vi "Template.Utility VI with Q Interface.vi"(7 "Q.Parent":refnum<queue>, 11 "Name":string) -> ()   [LabVIEW 2018]
uses:
  <vilib>/KATE/Queues/Q.Element.ctl
  <vilib>/KATE/Queues/Queue Utils.lvlib
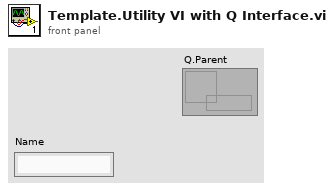
[diagram p1: front panel]
types:
  T1 = cluster{"Q.Parent":refnum<queue>, "Data1":bool, "Data2":string}
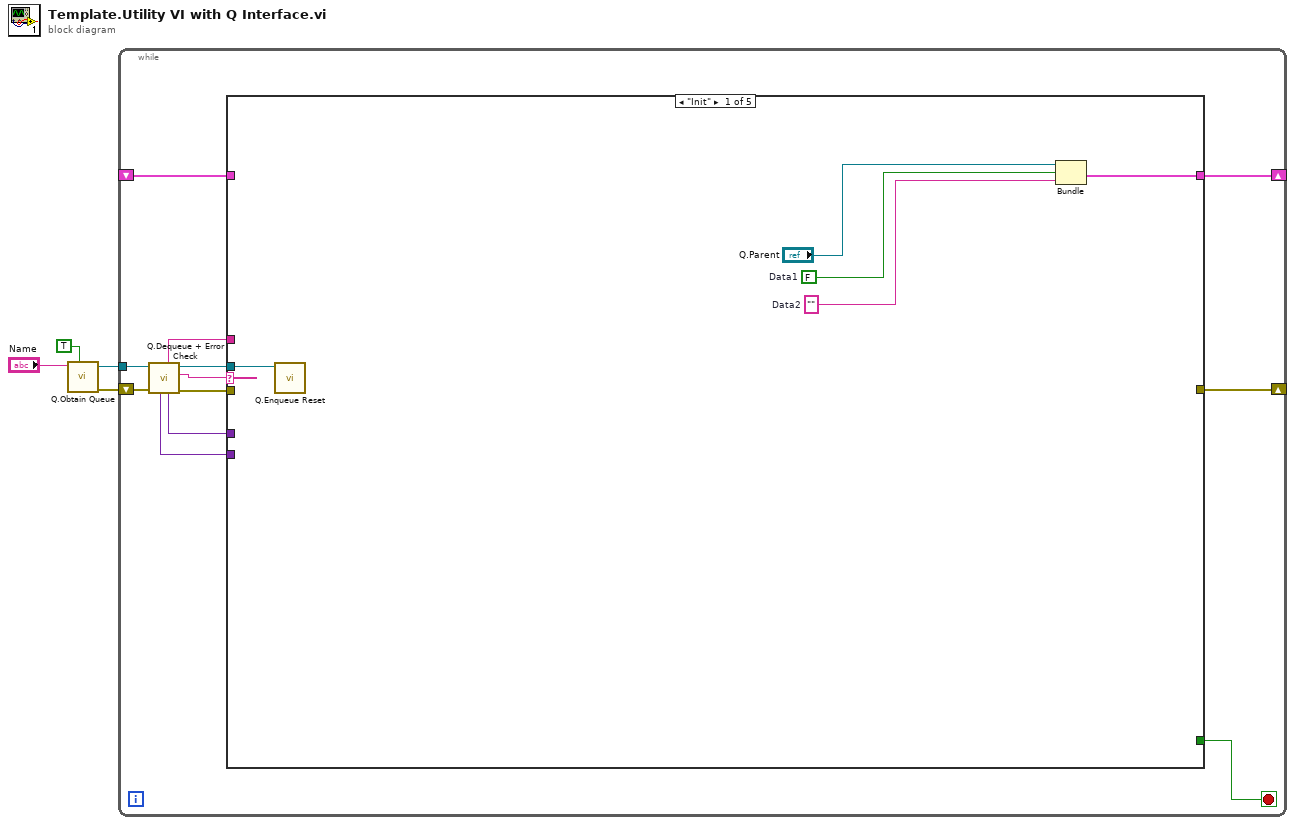
[diagram p0: block diagram]
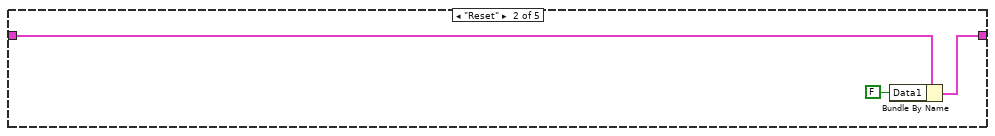
[diagram p2: hidden frame]
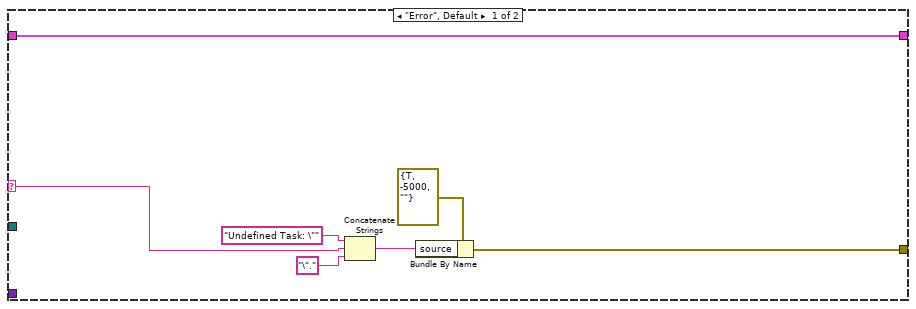
[diagram p4: hidden frame]
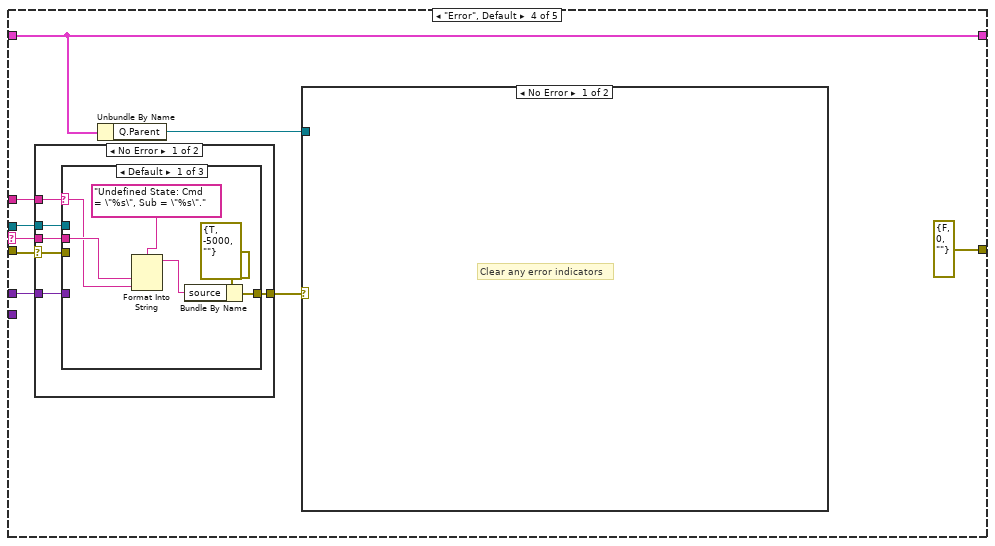
[diagram p5: hidden frame]
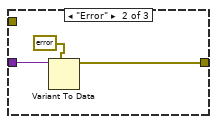
[diagram p6: hidden frame]
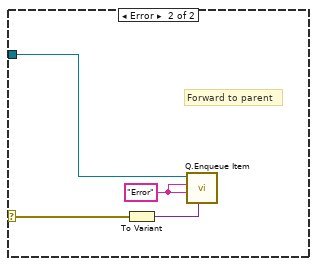
[diagram p9: hidden frame]
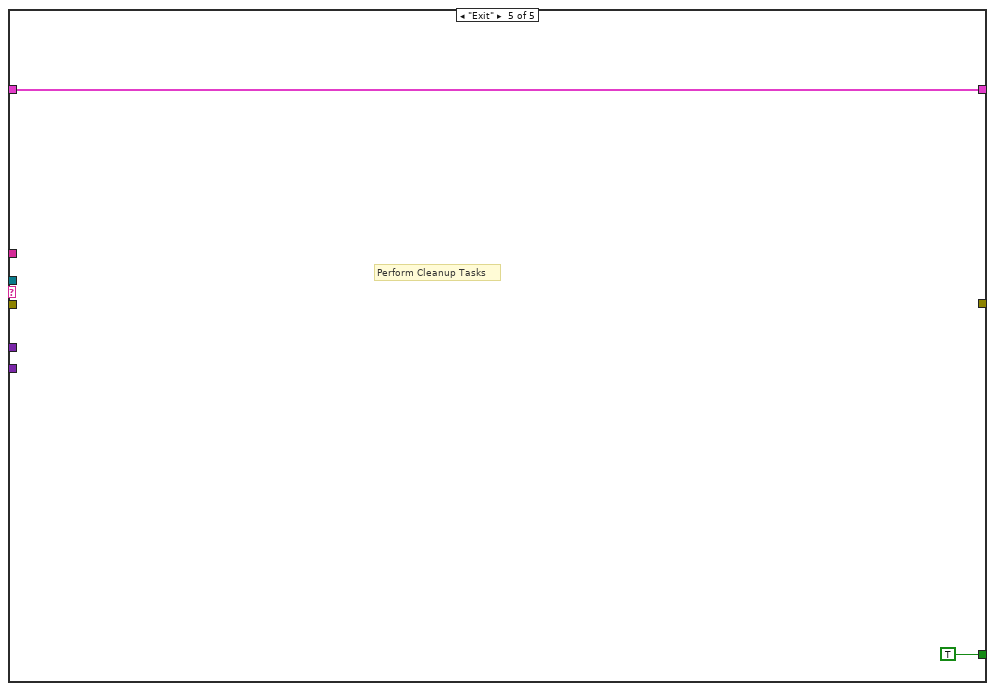
[diagram p10: hidden frame]
diagram:
  n1 = call <vilib>:"Q.Obtain Queue.vi"("Enqueue Init"=TRUE, "Q Name"="Name") -> ("error out"=w2:errorcluster, "Q Out"=w3:refnum<queue>)  [unwired: 7 in, 1 out]
  n2 = while {
    tunnel: w3 -> [w16]
    shift-right: [w6] -> _
    shift-left: w2 -> [w13]
    shift-right: [w7] -> _
    shift-left: _ -> [w8]
    stop <- w5 stop-if-true
    n3 = call <vilib>:"Q.Dequeue + Error Check.vi"("Error In"=w13, "Q In"=w16) -> ("error out"=w12:errorcluster, "Cmd"=w11:string, "Q Out"=w14:refnum<queue>, "Data1"=w10:variant, "Sub"=w15:string, "Data2"=w9:variant)  [unwired: 4 in]
    n4 = case shown="\"Init\"" w11 {
      selector: w11 -> [_ _ _ w40 _]
      tunnel: w15 -> [_ _ w30 w48 _]
      tunnel: w14 -> [w17 _ w29 w47 _]
      tunnel: w12 -> [_ _ _ w41 _]
      tunnel: w10 -> [_ _ w28 w46 _]
      tunnel: w9 -> [_ _ w27 _ _]
      tunnel: w8 -> [_ w24 w31 w44 w70]
      tunnel: [w19 w23 w26 w44 w70] -> w7
      tunnel: [_ _ w25 errorcluster {"status"=FALSE, "code"=0, "source"=""} ("error constant") _] -> w6
      tunnel: [_ _ _ _ TRUE] -> w5
      frame "Init" {
        w20 = ""  # Data2
        w21 = FALSE  # Data1
        n5 = call <vilib>:"Q.Enqueue Reset.vi"("Q In"=w17) -> ()  [unwired: 9 in, 2 out]
        n6 = Bundle("Q.Parent"="Q.Parent", "Data1"=w21, "Data2"=w20) -> (w19:T1)  [unwired: 1 in]
      }
      frame "Reset" {
        n7 = Bundle By Name(cluster=w24, "Data1"=FALSE) -> (w23:T1)
      }
      frame "Task" {
        n8 = case shown="\"XXX\"" w30 {
          selector: w30 -> [w33 _]
          tunnel: w31 -> [w38 w39]
          tunnel: w29 -> [_ _]
          tunnel: w28 -> [_ _]
          tunnel: w27 -> [_ _]
          tunnel: [w38 w39] -> w26
          tunnel: [w32 _] -> w25
          frame "Error", Default {
            n9 = Concatenate Strings("Undefined Task: \"", w33, "\".") -> (w34:string)
            n10 = Bundle By Name(cluster=errorcluster {"status"=TRUE, "code"=-5000, "source"=""} ("error constant"), "source"=w34) -> (w32:errorcluster)
          }
          frame "XXX" {
          }
        }
      }
      frame "Error", Default {
        n11 = case shown="No Error" w41 {
          selector: w41 -> [w50 w64]
          tunnel: w48 -> [w54 _]
          tunnel: w47 -> [w53 _]
          tunnel: w46 -> [w52 _]
          tunnel: [w51 w64] -> w45
          tunnel: w40 -> [w49 _]
          frame No Error {
            n12 = case shown="Default" w54 {
              selector: w54 -> [w59 _ _]
              tunnel: w52 -> [_ w63 _]
              tunnel: [w55 w61 _] -> w51
              tunnel: w53 -> [_ _ _]
              tunnel: w50 -> [_ _ _]
              tunnel: w49 -> [w60 _ _]
              frame Default {
                n13 = Format Into String(format string="Undefined State: Cmd = \"%s\", Sub = \"%s\".", w60, w59) -> (resulting string=w56:string)  [unwired: 2 in, 1 out]
                n14 = Bundle By Name(cluster=errorcluster {"status"=TRUE, "code"=-5000, "source"=""} ("error constant"), "source"=w56) -> (w55:errorcluster)
              }
              frame "Error" {
                n15 = Variant To Data(type=errorcluster {"status"=FALSE, "code"=0, "source"=""} ("error constant"), Variant=w63) -> (data=w61:errorcluster)  [unwired: 1 in, 1 out]
              }
              frame "Clear" {
              }
            }
          }
          frame Error {
          }
        }
        n16 = Unbundle By Name(w44) -> ("Q.Parent"=w43:refnum<queue>)
        n17 = case shown="No Error" w45 {
          selector: w45 -> [_ w66]
          tunnel: w43 -> [_ w65]
          frame No Error {
            # "Clear any error indicators"
          }
          frame Error {
            w67 = "Error"
            # "Forward to parent"
            n18 = To Variant(anything=w66) -> (Variant=w68:variant)
            n19 = call <vilib>:"Q.Enqueue Item.vi"("Data1"=w68, "Sub"=w67, "Cmd"=w67, "Q In"=w65) -> ()  [unwired: 6 in, 2 out]
          }
        }
      }
      frame "Exit" {
        # "Perform Cleanup Tasks"
      }
    }
  }
